vi "MT_RT_EQC.vi"(9 "Data":i32, 10 "Qty":i32, 11 "input string":string) -> (0 "EQC":i32, 1 "RT":i32, 2 "Station":string, 3 "MT":i32, 4 "STN":string)   [LabVIEW 2012]
uses:
  <vilib>/regexp/Match Regular Expression.xnode
panel:
  out "all upper case string":string
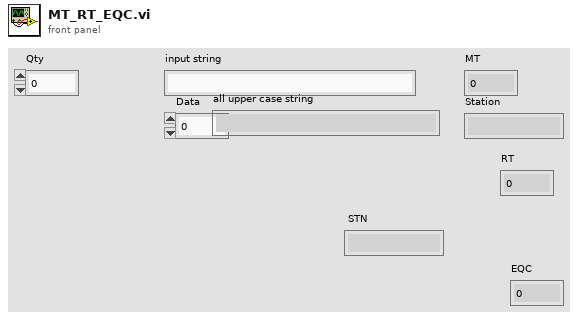
[diagram p1: front panel]
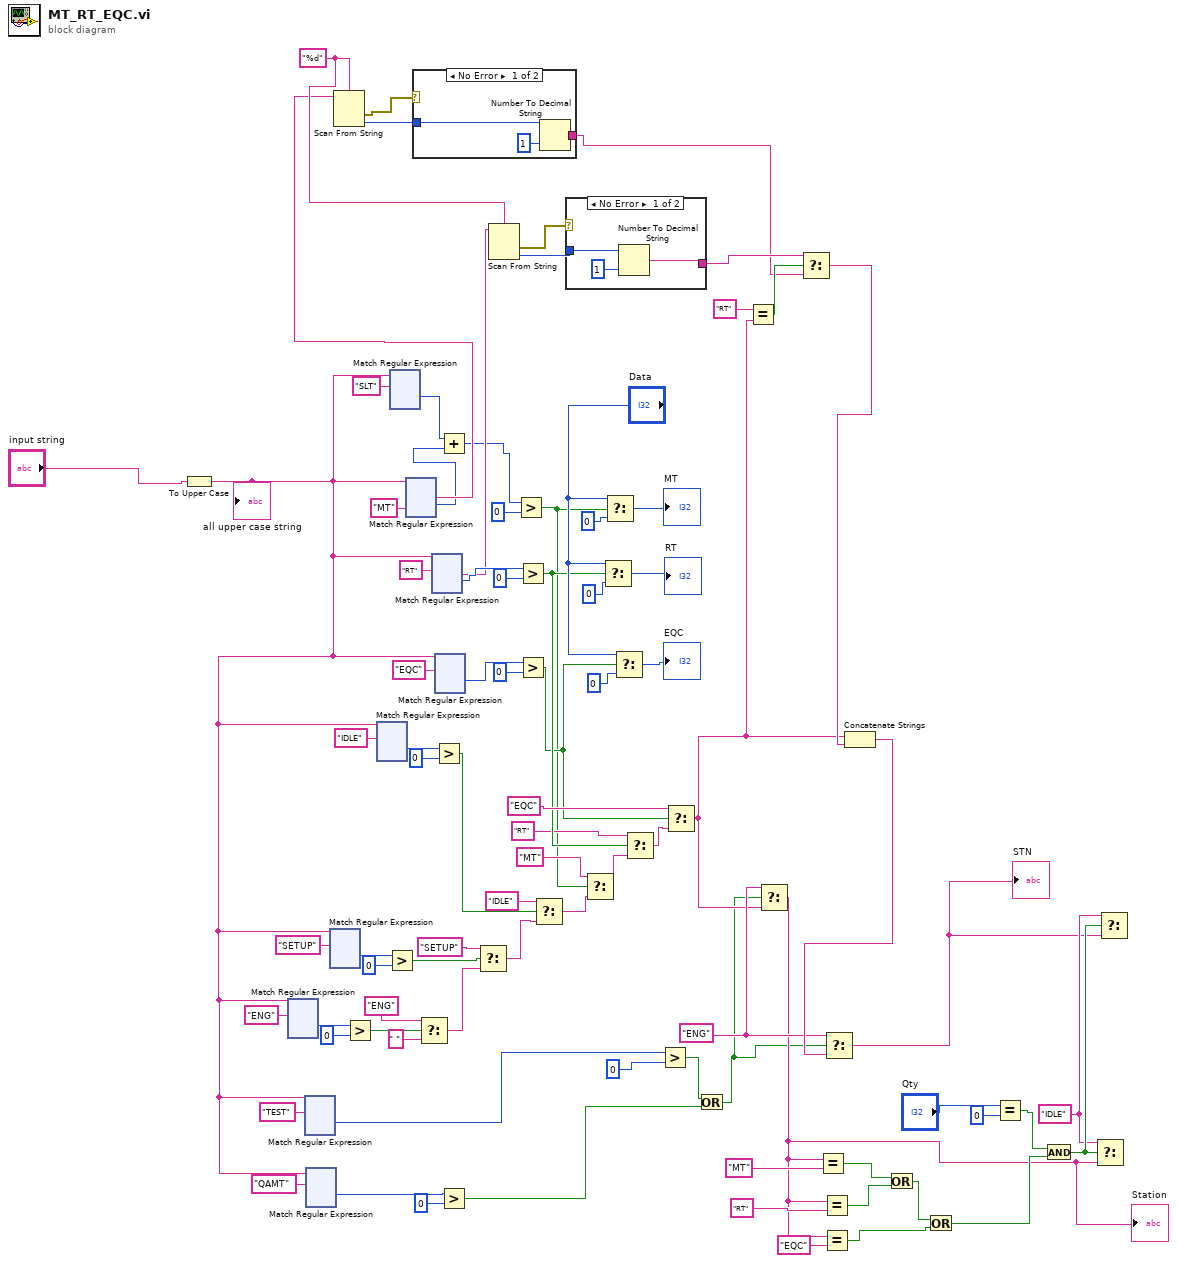
[diagram p0: block diagram]
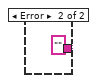
[diagram p2: hidden frame]
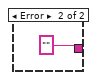
[diagram p3: hidden frame]
diagram:
  w14 = "IDLE" ("t")
  w28 = "ENG" ("t")
  w43 = "%d" ("format string")
  n1 = To Upper Case(1:"input string") -> (0:w5:string)
  "all upper case string" <- w5
  n2 = xnode "Match Regular Expression"("input string"=w5, "regular expression"="ENG") -> ("offset past match"=w51:i32)  [unwired: 4 in, 4 out]
  n3 = xnode "Match Regular Expression"("input string"=w5, "regular expression"="TEST") -> ("offset past match"=w31:i32)  [unwired: 4 in, 4 out]
  n4 = xnode "Match Regular Expression"("input string"=w5, "regular expression"="QAMT") -> ("offset past match"=w10:i32)  [unwired: 4 in, 4 out]
  n5 = xnode "Match Regular Expression"("input string"=w5, "regular expression"="SETUP") -> ("offset past match"=w57:i32)  [unwired: 4 in, 4 out]
  n6 = Greater?(x=w51, y=0) -> (0:w49:bool)
  n7 = xnode "Match Regular Expression"("input string"=w5, "regular expression"="IDLE") -> ("offset past match"=w65:i32)  [unwired: 4 in, 4 out]
  n8 = Greater?(x=w57, y=0) -> (0:w54:bool)
  n9 = xnode "Match Regular Expression"("input string"=w5, "regular expression"="SLT") -> ("offset past match"=w3:i32)  [unwired: 4 in, 4 out]
  n10 = xnode "Match Regular Expression"("input string"=w5, "regular expression"="MT") -> ("after match"=w36:string, "offset past match"=w2:i32)  [unwired: 4 in, 3 out]
  n11 = Scan From String(format string=w43, input string=w36) -> (error out=w44:errorcluster, output 1=w45:i32)  [unwired: 3 in, 2 out]
  n12 = case shown="No Error" w44 {
    tunnel: [w89 ""] -> w37
    tunnel: w45 -> [w88 _]
    frame No Error {
      n13 = Number To Decimal String(number=w88, width (-)=i16 1) -> (decimal integer string=w89:string)
    }
    frame Error {
    }
  }
  n14 = Select(t="ENG", s=w49, f=" ") -> (s? t:f=w48:string)
  n15 = xnode "Match Regular Expression"("input string"=w5, "regular expression"="RT") -> ("after match"=w35:string, "offset past match"=w81:i32)  [unwired: 4 in, 3 out]
  n16 = Greater?(x=w65, y=0) -> (0:w62:bool)
  n17 = xnode "Match Regular Expression"("input string"=w5, "regular expression"="EQC") -> ("offset past match"=w80:i32)  [unwired: 4 in, 4 out]
  n18 = Add(x=w3, y=w2) -> (x+y=w1:i32)
  n19 = Greater?(x=w10, y=0) -> (0:w6:bool)
  n20 = Select(t="SETUP", s=w54, f=w48) -> (s? t:f=w53:string)
  n21 = Scan From String(format string=w43, input string=w35) -> (error out=w42:errorcluster, output 1=w41:i32)  [unwired: 3 in, 2 out]
  n22 = Greater?(x=w1, y=0) -> (0:w59:bool)
  n23 = Greater?(x=w81, y=0) -> (0:w70:bool)
  n24 = Greater?(x=w80, y=0) -> (0:w60:bool)
  n25 = Select(t="IDLE", s=w62, f=w53) -> (s? t:f=w63:string)
  n26 = case shown="No Error" w42 {
    tunnel: [w92 ""] -> w38
    tunnel: w41 -> [w93 _]
    frame No Error {
      n27 = Number To Decimal String(number=w93, width (-)=i16 1) -> (decimal integer string=w92:string)
    }
    frame Error {
    }
  }
  n28 = Select(t="MT" ("f"), s=w59, f=w63) -> (s? t:f=w68:string)
  n29 = Select(t="Data", s=w70, f=0) -> (s? t:f=→"RT":i32)
  n30 = Select(t="Data", s=w59, f=0) -> (s? t:f=→"MT":i32)
  n31 = Select(t="Data", s=w60, f=0) -> (s? t:f=→"EQC":i32)
  n32 = Select(t="RT" ("f"), s=w70, f=w68) -> (s? t:f=w71:string)
  n33 = Greater?(x=w31, y=0) -> (0:w7:bool)
  n34 = Select(t="EQC", s=w60, f=w71) -> (s? t:f=w27:string)
  n35 = Or(x=w7, y=w6) -> (x .or. y?=w8:bool)
  n36 = Equal?(x="RT", y=w27) -> (x = y?=w39:bool)
  n37 = Select(t=w28, s=w8, f=w27) -> (s? t:f=w12:string)
  "Station" <- w12
  n38 = Select(t=w38, s=w39, f=w37) -> (s? t:f=w34:string)
  n39 = Equal?(x=w12, y="MT") -> (x = y?=w21:bool)
  n40 = Equal?(x=w12, y="RT") -> (x = y?=w20:bool)
  n41 = Equal?(x=w12, y="EQC") -> (x = y?=w18:bool)
  n42 = Concatenate Strings(w27, w34) -> (w29:string)
  n43 = Select(t=w28, s=w8, f=w29) -> (s? t:f=w13:string)
  "STN" <- w13
  n44 = Or(x=w21, y=w20) -> (x .or. y?=w19:bool)
  n45 = Or(x=w19, y=w18) -> (x .or. y?=w16:bool)
  n46 = Equal?(x="Qty", y=0) -> (x = y?=w17:bool)
  n47 = And(x=w17, y=w16) -> (x .and. y?=w15:bool)
  n48 = Select(t=w14, s=w15, f=w12) -> ()  [unwired: 1 out]
  n49 = Select(t=w14, s=w15, f=w13) -> ()  [unwired: 1 out]
